vi "Add triggered Events.vi"(9 "Triggers":bool[](array[boolean]), 10 "States  List":string[](array[string]), 11 "List In":string[](array[string])) -> (3 "List Out":string[](array[string]))   [LabVIEW 2018]
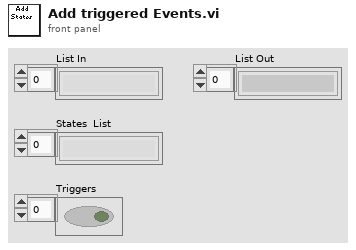
[diagram p1: front panel]
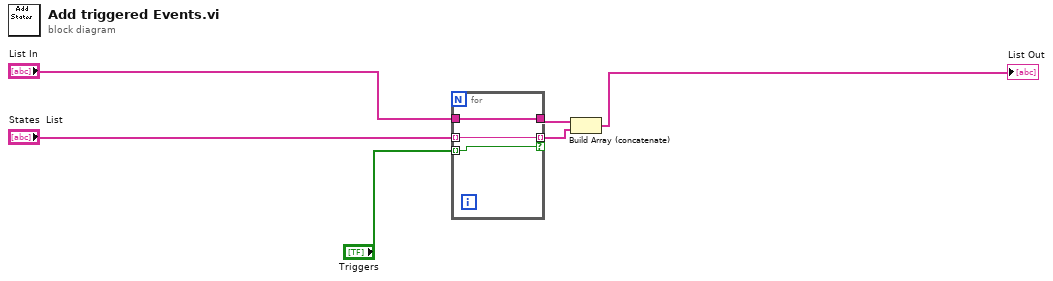
[diagram p0: block diagram]
diagram:
  n1 = for {
    tunnel: "States  List" -> [w9] mode=indexing
    tunnel: "Triggers" -> [w8] mode=indexing
    tunnel: [w9] -> w5 mode=indexing if=w8
    tunnel: "List In" -> [w7]
    tunnel: [w7] -> w4
  }
  n2 = Build Array (concatenate)(w4, w5) -> (→"List Out":string[])
